vi "GPIB_autodetect.vi"(7 "ID command":string, 8 "error in (no error)":errorcluster, 9 "Verify GPIB address":bool, 10 "Instrument address in":refnum<visa-resource-name>, 11 "InstrControl in":refnum<class "InstrControl.lvclass">) -> (0 "error out":errorcluster, 2 "Instrument address out":refnum<visa-resource-name>, 3 "InstrControl out":refnum<class "InstrControl.lvclass">)   [LabVIEW 2019, in "InstrControl.lvclass"]
uses:
  InstrControl.lvclass
panel:
  out "addresses found":string[](array[string])
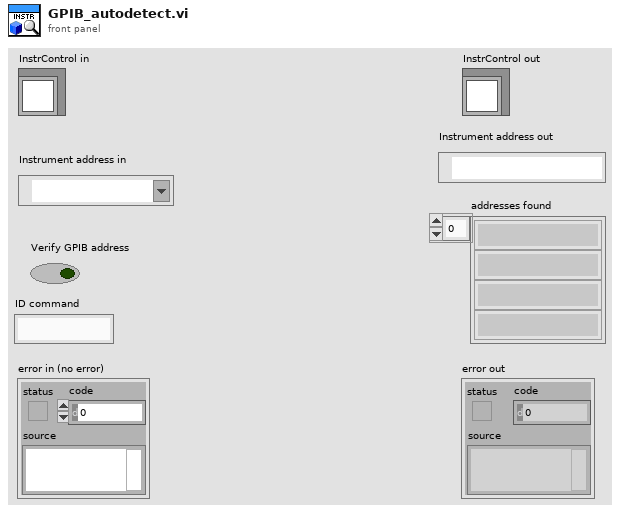
[diagram p1: front panel]
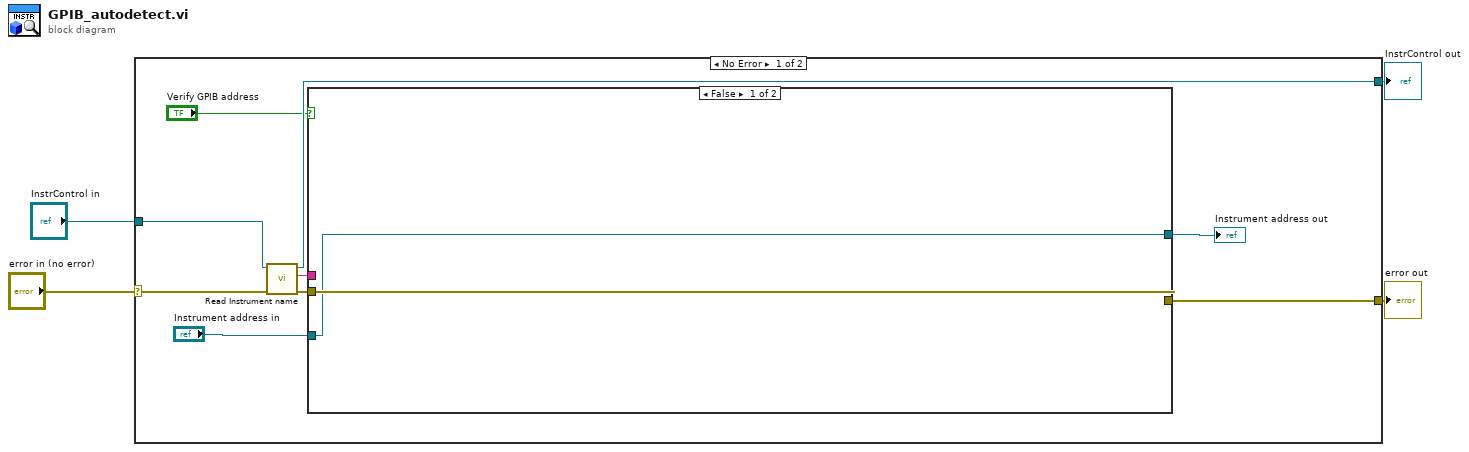
[diagram p0: block diagram]
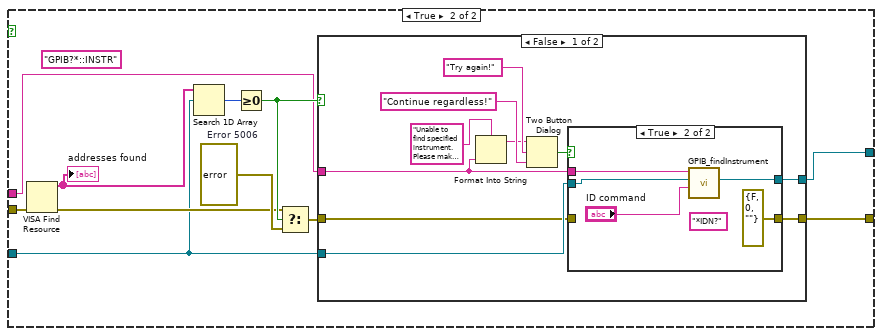
[diagram p2: hidden frame]
diagram:
  n1 = case shown="No Error" "error in (no error)" {
    selector: "error in (no error)" -> [w12 w47]
    tunnel: [w9 w47] -> w3
    tunnel: [w11 w46] -> w1
    tunnel: "InstrControl in" -> [w13 w46]
    frame No Error {
      n2 = call-dynamic "Read Instrument name.vi"("error in (no error)"=w12, "InstControl in"=w13) -> ("error out"=w10:errorcluster, "Instrument name"=w8:string, "InstControl out"=w11:refnum<class "InstrControl.lvclass">)  [unwired: 7 in]
      n3 = case shown="False" "Verify GPIB address" {
        tunnel: w10 -> [w15 w25]
        tunnel: [w15 w21] -> w9
        tunnel: w8 -> [_ w20]
        tunnel: "Instrument address in" -> [w14 w17]
        tunnel: [w14 w16] -> w5
        frame False {
        }
        frame True {
          w26 = errorcluster {"status"=FALSE, "code"=5005, "source"="Unable to find specified instrument.  Please make sure the it is connected to your system and switched on."}  # Error 5006
          (unwired) "GPIB?*::INSTR" ("expression (\"\")")
          n4 = VISA Find Resource(8:w25) -> (0:w18:errorcluster, 3:w19:string[])  [unwired: 2 in, 1 out]
          "addresses found" <- w19
          n5 = Search 1D Array(1D array=w19, element=w17) -> (index of element=w24:i32)  [unwired: 1 in]
          n6 = Greater Or Equal To 0?(x=w24) -> (x >= 0?=w23:bool)
          n7 = Select(t=w18, s=w23, f=w26) -> (s? t:f=w22:errorcluster)
          n8 = case shown="False" w23 {
            tunnel: w17 -> [w33 w45]
            tunnel: [w32 w45] -> w16
            tunnel: w22 -> [w31 w44]
            tunnel: [w30 w44] -> w21
            tunnel: w20 -> [w28 _]
            frame False {
              n9 = Format Into String(format string="Unable to find specified instrument.  Please make sure the it is connected to your system and switched on.\n\n%s" ("source"), w28) -> (resulting string=w27:string)  [unwired: 2 in, 1 out]
              n10 = Two Button Dialog(message=w27, 1:"Continue regardless!", 2:"Try again!") -> (T button?=w34:bool)
              n11 = case shown="True" w34 {
                tunnel: w33 -> [w38 w43]
                tunnel: [w38 w42] -> w32
                tunnel: w31 -> [w37 _]
                tunnel: [w37 errorcluster {"status"=FALSE, "code"=0, "source"=""} ("error constant")] -> w30
                tunnel: w28 -> [_ w40]
                frame False {
                }
                frame True {
                  (unwired) "*IDN?" ("regular expression")
                  n12 = call "GPIB_findInstrument.vi"("ID command"="ID command", "revised Instrument address"=w43, "Instrument name IN"=w40) -> ("revised GPIB address OUT"=w42:refnum<visa-resource-name>)  [unwired: 8 in]
                }
              }
            }
            frame True {
            }
          }
        }
      }
      "Instrument address out" <- w5
    }
    frame Error {
    }
  }
  "error out" <- w3
  "InstrControl out" <- w1
